vi "coupling_magnitude.vi"(6 "Carrier sense":cdb[](array[numeric]), 10 "Carrier amplitudes":cdb[][][](array[numeric]), 11 "Output options":T1) -> (3 "Magnitudes":dbl[](array[numeric]))   [LabVIEW 2014]
uses:
  output_options.ctl
  coupling_selector.ctl
panel:
  # "Coupling magnitude across time"
  # "Time sample"
  # "XYZ carrier"
  # "XYZ in channel"
  # "X"
  # "Carrier"
  # "Y"
  # "Z"
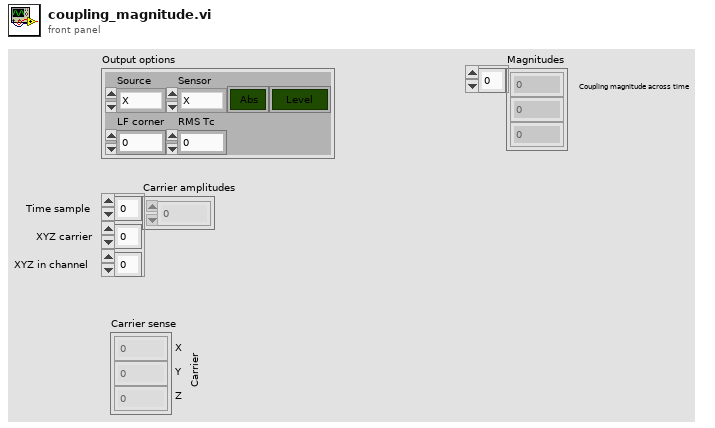
[diagram p1: front panel]
types:
  T1 = typedef "output_options.ctl" = cluster{"Source":T2, "Sensor":T2, "Sense":bool, "Distance":bool, "LF corner":dbl, "RMS Tc":dbl}
  T2 = typedef "coupling_selector.ctl" = enum16{"X", "Y", "Z", "Vector"}
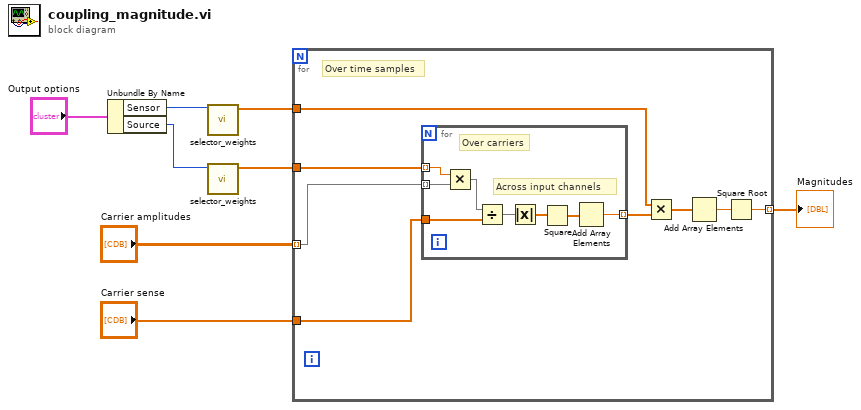
[diagram p0: block diagram]
diagram:
  n1 = Unbundle By Name("Output options") -> ("Sensor"=w3:T2, "Source"=w4:T2)
  n2 = call "selector_weights.vi"("Selector"=w3) -> ("Weights"=w6:dbl[])  [unwired: 10 in]
  n3 = call "selector_weights.vi"("Selector"=w4) -> ("Weights"=w5:dbl[])  [unwired: 10 in]
  n4 = for {
    tunnel: "Carrier amplitudes" -> [w16] mode=indexing
    tunnel: "Carrier sense" -> [w15]
    tunnel: w5 -> [w12]
    tunnel: w6 -> [w13]
    tunnel: [w11] -> w1 mode=indexing
    # "Over time samples"
    n5 = for {
      tunnel: w16 -> [w18] mode=indexing
      tunnel: w15 -> [w24]
      tunnel: [w20] -> w14 mode=indexing
      tunnel: w12 -> [w19] mode=indexing
      # "Across input channels"
      # "Over carriers"
      n6 = Multiply(x=w19, y=w18) -> (x*y=w17:cdb[])
      n7 = Divide(x=w17, y=w24) -> (x/y=w21:cdb[])
      n8 = Absolute Value(x=w21) -> (abs(x)=w23:dbl[])
      n9 = Square(x=w23) -> (x^2=w22:dbl[])
      n10 = Add Array Elements(numeric array=w22) -> (sum=w20:dbl)
    }
    n11 = Multiply(x=w13, y=w14) -> (x*y=w10:dbl[])
    n12 = Add Array Elements(numeric array=w10) -> (sum=w9:dbl)
    n13 = Square Root(x=w9) -> (sqrt(x)=w11:dbl)
  }
  "Magnitudes" <- w1
